vi "TestGetProjectConditionalDeactivationValues.vi"(11 "Key":string) -> (0 "Fehler (Ausgang)":errorcluster, 3 "Value":string, 5 "Values":string[](array[string]), 7 "Keys":string[](array[string]))   [LabVIEW 2015, in "ConditionalDeactivation.lvlib"]
uses:
  ConditionalDeactivation.lvlib
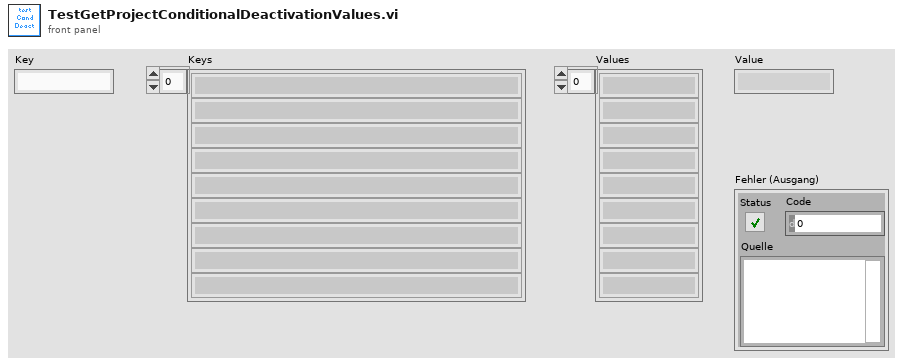
[diagram p1: front panel]
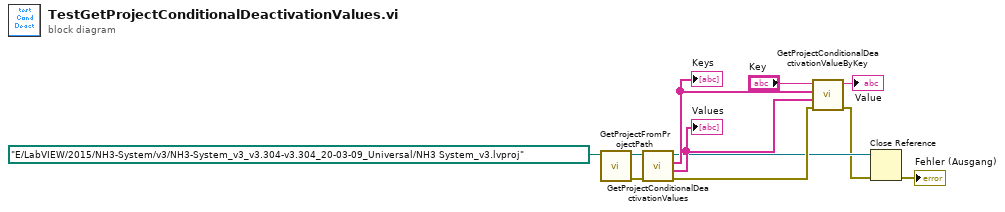
[diagram p0: block diagram]
diagram:
  n1 = call "GetProjectFromProjectPath.vi"("ProjectPfad"=path "E:/LabVIEW/2015/NH3-System/v3/NH3-System_v3_v3.304-v3.304_20-03-09_Universal/NH3 System_v3.lvproj") -> ("Fehler (Ausgang)"=w9:errorcluster, "Projekt Referenz"=w10:refnum<vi>)  [unwired: 9 in]
  n2 = call "GetProjectConditionalDeactivationValues.vi"("Fehler (Eingang, kein Fehler)"=w9, "Projekt Referenz"=w10) -> ("Fehler (Ausgang)"=w6:errorcluster, "Values"=w7:string[], "Keys"=w8:string[], "Projekt Referenz"=w3:refnum<vi>)  [unwired: 5 in, 1 out]
  "Keys" <- w8
  "Values" <- w7
  n3 = call "GetProjectConditionalDeactivationValueByKey.vi"("Fehler (Eingang, kein Fehler)"=w6, "Values"=w7, "Keys"=w8, "Key"="Key") -> ("Fehler (Ausgang)"=w2:errorcluster, "Value out"=→"Value":string)  [unwired: 3 in, 3 out]
  n4 = Close Reference(reference=w3, error in (no error)=w2) -> (error out=→"Fehler (Ausgang)":errorcluster)
